vi "Set_Symbols.vi"(8 "error in (no error)":errorcluster, 11 "IB_Tree in":refnum<class "IB_Tree.lvclass">) -> (0 "error out":errorcluster, 3 "IB_Tree out":refnum<class "IB_Tree.lvclass">)   [LabVIEW 2020, in "IB_Tree.lvclass"]
uses:
  <vilib>/AppBuilder/IB_Classes/Tree/IB_Tree.lvclass
  <vilib>/AppBuilder/IB_Classes/Tree/IB_Tree.lvclass/IB_Tree.ctl
  <resource>/Framework/Providers/Builds/Installer/SRdB_Icon/SRdB_Icon_action.ctl
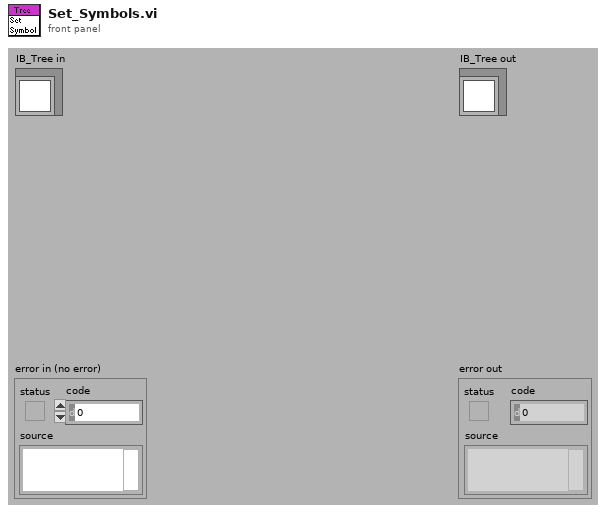
[diagram p1: front panel]
types:
  T1 = typedef "SRdB_Icon_action.ctl" = enum16{"read", "write", "create", "delete", "initialize", "unInitialize", "getLock", "readAll", "writeAll"}
  T2 = typedef "SRdB_Icon.ctl" = cluster{"extension":string, "image data":T3}
  T3 = typedef "imagedata.ctl" = cluster{"image type":i32, "image depth":i32, "image":u8[], "mask":u8[], "colors":u32[], "Rectangle":cluster{"left":i16, "top":i16, "right":i16, "bottom":i16}}
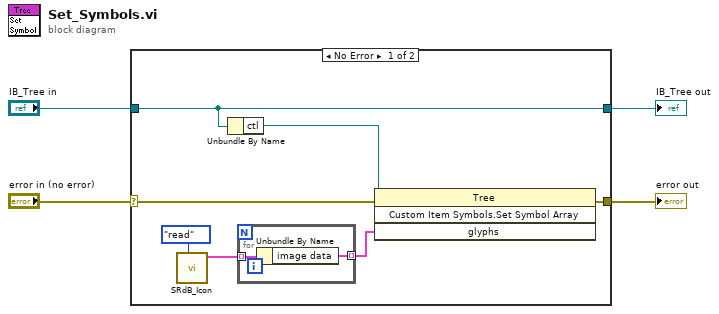
[diagram p0: block diagram]
diagram:
  n1 = case shown="No Error" "error in (no error)" {
    selector: "error in (no error)" -> [w9 w15]
    tunnel: [w8 w15] -> w3
    tunnel: [w11 w14] -> w1
    tunnel: "IB_Tree in" -> [w11 w14]
    frame No Error {
      n2 = call <resource>:"SRdB_Icon.vi"("action"=SRdB_Icon_action."read") -> ("icons"=w6:T2[])  [unwired: 8 in, 2 out]
      n3 = Unbundle By Name(w11) -> ("ctl"=w10:refnum<vi>)
      n4 = for {
        tunnel: w6 -> [w13] mode=indexing
        tunnel: [w12] -> w5 mode=indexing
        n5 = Unbundle By Name(w13) -> ("image data"=w12:T3)
      }
      n6 = invoke class="Tree" method="Custom Item Symbols.Set Symbol Array"(reference=w10, error in=w9, "glyphs"=w5) -> (error out=w8:errorcluster)  [unwired: 1 in, 3 out]
    }
    frame Error {
    }
  }
  "error out" <- w3
  "IB_Tree out" <- w1
